vi "Create Single Pixel ROIs from ROI (Core).vi"(5 "Y Resolution":i32, 7 "X Resolution":i32, 8 "error in (no error)":errorcluster, 11 "ROI Descriptor":T1 {"Contours"."Type" items=["No Selection", "Point", "Line", "Rectangle", "Oval", "Polygon", "Freehand Region", "Annulus", "Unused2", "Unused3", "Broken Line", "Freehand Line", "Rotated Rectangle"]}) -> (0 "error out":errorcluster, 2 "Aborted":bool, 3 "Point Array":cluster{"Numeric":i32, "Numeric":i32}[](array[cluster]))   [LabVIEW 2021, in "Image.lvlib"]
uses:
  Image.lvlib
  Abort ROI Creation Global.vi
  <vilib>/vision/NI_Vision_Development_Module.lvlib
  Utilities/Utilities.lvlib
  Error/Error.lvlib
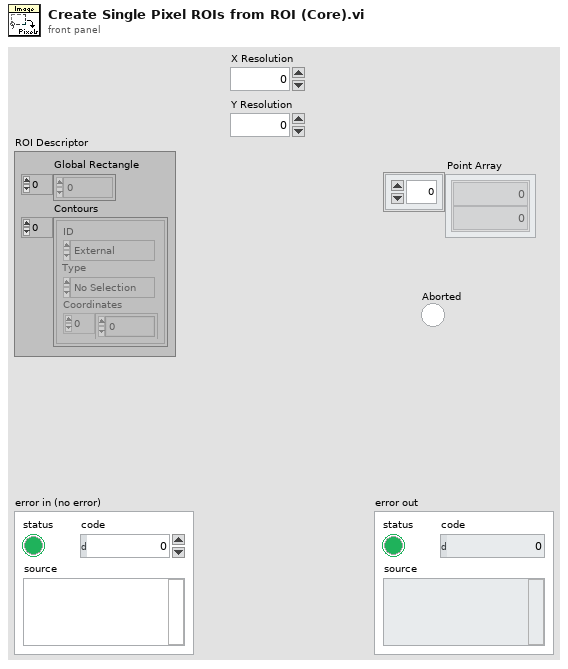
[diagram p1: front panel]
types:
  T1 = typedef "ROI Descriptor" = cluster{"Global Rectangle":i32[], "Contours":cluster{"ID":enum32{"External", "Internal"}, "Type":u32, "Coordinates":i32[]}[]}
  T2 = typedef "Image Type" = u32
  T3 = typedef "IMAQ Image.ctl" = refnum<image>
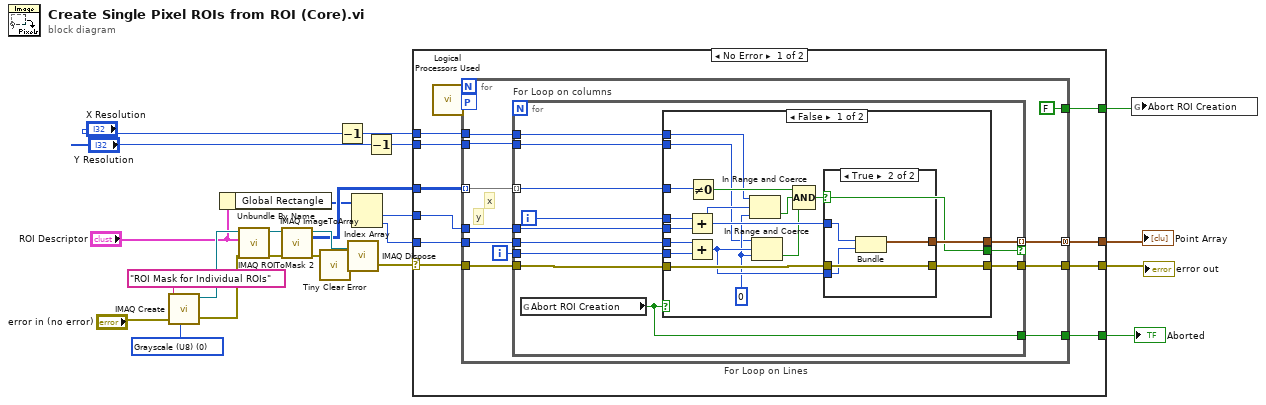
[diagram p0: block diagram]
diagram:
  w6 = T2 0 items=["Grayscale (U8)", "Grayscale (I16)", "Grayscale (SGL)", "Complex (CSG)", "RGB (U32)", "HSL (U32)", "RGB (U64)", "Grayscale (U16)"] ("Image Type")
  n1 = call "IMAQ Create"("Image Name"="ROI Mask for Individual ROIs", "Image Type"=w6, "error in (no error)"="error in (no error)") -> ("New Image"=w5:T3, "error out"=w23:errorcluster)  [unwired: 2 in]
  n2 = Unbundle By Name("ROI Descriptor") -> ("Global Rectangle"=w9:i32[])
  n3 = call "IMAQ ROIToMask 2"("error in (no error)"=w23, "ROI Descriptor"="ROI Descriptor", "Image"=w5) -> ("error out"=w8:errorcluster, "Image Out"=w15:T3)  [unwired: 6 in, 1 out]
  n4 = call "IMAQ ImageToArray"("error in (no error)"=w8, "Image"=w15) -> ("error out"=w14:errorcluster, "Image Pixels (U8)"=w10:u8[][])  [unwired: 2 in, 3 out]
  n5 = call "Tiny Clear Error.vi"("Error In"=w14) -> ("no Error Out"=w1:errorcluster)  [unwired: 8 in]
  n6 = Decrement(x="X Resolution") -> (x-1=w17:i32)
  n7 = call "IMAQ Dispose"("Image"=w15, "error in (no error)"=w1) -> ("error out"=w20:errorcluster)  [unwired: 4 in]
  n8 = Index Array(array=w9) -> (element #1=w11:i32, element #2=w12:i32)  [unwired: 2 in]
  n9 = Decrement(x="Y Resolution") -> (x-1=w19:i32)
  n10 = case shown="No Error" w20 {
    selector: w20 -> [w32 w80]
    tunnel: [w34 _] -> w21
    tunnel: w19 -> [w31 _]
    tunnel: w17 -> [w30 _]
    tunnel: [w29 _] -> w13
    tunnel: w12 -> [w28 _]
    tunnel: w11 -> [w27 _]
    tunnel: w10 -> [w26 _]
    tunnel: [w25 _] -> w3
    tunnel: [w24 w80] -> w2
    frame No Error {
      n11 = call "Logical Processors Used.vi"() -> ("# Logical Processor Used"=w33:i32)  [unwired: 6 in]
      n12 = for "For Loop on Lines" {
        tunnel: w26 -> [w45] mode=indexing
        tunnel: w28 -> [w44]
        tunnel: w27 -> [w43]
        tunnel: [w42] -> w29 mode=concatenating
        tunnel: w30 -> [w38]
        tunnel: w31 -> [w37]
        tunnel: w32 -> [w41]
        tunnel: [w40] -> w24
        workers-P: w33 -> [_]
        tunnel: [w36] -> w34
        tunnel: [FALSE ("Abort ROI Creation")] -> w25
        i -> [w39]
        # "x"
        # "y"
        n13 = for "For Loop on columns" {
          tunnel: w45 -> [w57] mode=indexing
          tunnel: w44 -> [w50]
          tunnel: w43 -> [w52]
          tunnel: [w56] -> w42 mode=indexing if=w47
          tunnel: w39 -> [w51]
          tunnel: w38 -> [w49]
          tunnel: w37 -> [w48]
          tunnel: w41 -> [w55]
          tunnel: [w54] -> w40
          tunnel: [w46] -> w36
          i -> [w53]
          n14 = global read "Abort ROI Creation Global.vi" "Abort ROI Creation"() -> (w46:bool)
          n15 = case shown="False" w46 {
            tunnel: w57 -> [w74 _]
            tunnel: [w73 _] -> w56
            tunnel: w55 -> [w71 _]
            tunnel: [w70 _] -> w54
            tunnel: w53 -> [w69 _]
            tunnel: w52 -> [w68 _]
            tunnel: w51 -> [w67 _]
            tunnel: w50 -> [w66 _]
            tunnel: [w60 _] -> w47
            tunnel: w49 -> [w59 _]
            tunnel: w48 -> [w58 _]
            frame False {
              w62 = 0 ("lower limit")
              n16 = Add(x=w69, y=w68) -> (x+y=w65:i32)
              n17 = Add(x=w66, y=w67) -> (x+y=w63:i32)
              n18 = Not Equal To 0?(x=w74) -> (x != 0?=w72:bool)
              n19 = In Range and Coerce(upper limit=w59, x=w65, lower limit=w62) -> (In Range?=w64:bool)  [unwired: 1 out]
              n20 = In Range and Coerce(upper limit=w58, x=w63, lower limit=w62) -> (In Range?=w61:bool)  [unwired: 1 out]
              n21 = Compound Arithmetic op=AND(w72, w64, w61) -> (w60:bool)
              n22 = case shown="True" w60 {
                tunnel: w65 -> [_ w78]
                tunnel: w63 -> [_ w77]
                tunnel: [_ w76] -> w73
                tunnel: w71 -> [w75 w79]
                tunnel: [w75 w79] -> w70
                frame False {
                }
                frame True {
                  n23 = Bundle(w78, w77) -> (w76:cluster{i32, i32})  [unwired: 1 in]
                }
              }
            }
            frame True {
            }
          }
        }
      }
    }
    frame Error {
    }
  }
  "error out" <- w2
  "Point Array" <- w13
  "Aborted" <- w21
  n24 = global write "Abort ROI Creation Global.vi" "Abort ROI Creation"(w3) -> ()
